vi "DiffDriveTrainSim_New_Mass_MOI.vi"(5 "j_KgM2":dbl=1.0, 6 "MeasurementStdDev":T1, 7 "Mass_Kg":dbl, 8 "WheelRadius_M":dbl, 9 "TrackWidth_M":dbl, 10 "Gearing":dbl=1.0, 11 "DriveMotor":T2 {"Kt_NMPerAmp" format="%13.5p"; "Kv_RadPerSecPerVolt" format="%13.5p"; "R_Ohms" format="%13.5p"; "FreeSpeed_RadPerSec" format="%13.5p"; "FreeCurrent_Amps" format="%13.5p"; "StallCurrent_Amps" format="%13.5p"; "StallTorque_NM" format="%13.5p"; "nominalVoltage_Volts" format="%13.5p"}) -> (0 "Size Coerced":bool, 3 "DiffDriveTrainSim":T3 {"m_Motor"."Kt_NMPerAmp" format="%13.5p"; "m_Motor"."Kv_RadPerSecPerVolt" format="%13.5p"; "m_Motor"."R_Ohms" format="%13.5p"; "m_Motor"."FreeSpeed_RadPerSec" format="%13.5p"; "m_Motor"."FreeCurrent_Amps" format="%13.5p"; "m_Motor"."StallCurrent_Amps" format="%13.5p"; "m_Motor"."StallTorque_NM" format="%13.5p"; "m_Motor"."nominalVoltage_Volts" format="%13.5p"})   [LabVIEW 2019, in "Trajectory_Library.lvlib"]
doc: "Creates a new LINEAR SYSTEM data cluster with the specified values. \n\n\nInputs: \n - XXX -- XXX.\n\nOutputs:\n - XXX -- XXX."
uses:
  Trajectory_Library.lvlib
  DIFF_DRIVE_TRAIN_SIM.ctl
  LINEAR_SYSTEM.ctl
  <vilib>/Analysis/Matrix/Datatypes/RealMatrix.ctl
  DCMOTOR.CTL
  MatBuilder_Create.vi
  MatBuilder_Fill.vi
  MatrixHelper_Zero.vi
  LinearSystem_New.vi
  <vilib>/Analysis/Matrix/NI_Matrix.lvlib
panel:
  # "<1, 1>"
  # "<States, 1>"
  # "<Outputs, 1>"
  # "<Inputs, 1>"
  # "<Outputs, 1>"
  # "<States,States>"
  # "<States,Inputs>"
  # "<Outputs,States>"
  # "<Outputs,Inputs>"
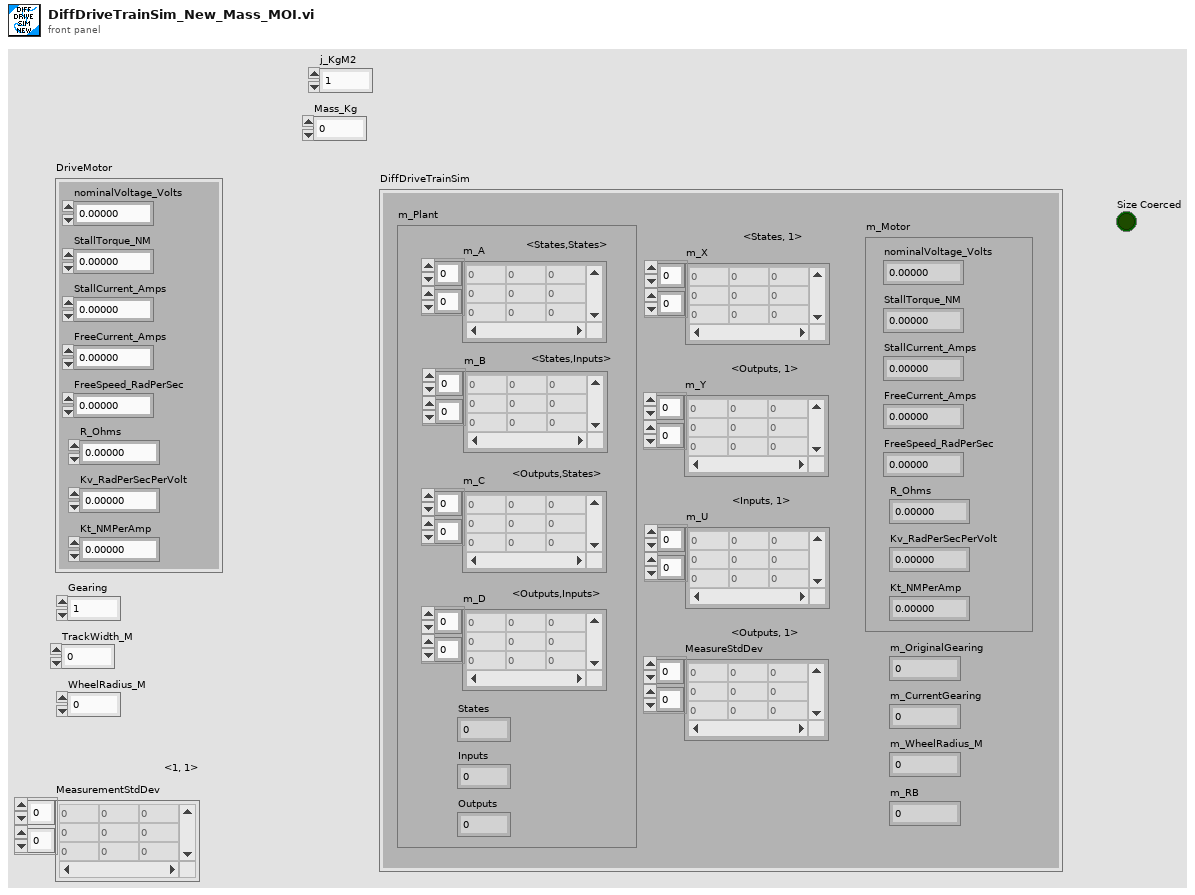
[diagram p1: front panel]
types:
  T1 = typedef "NI_Matrix.lvlib/RealMatrix.ctl" = dbl[][]
  T2 = typedef "Trajectory_Library.lvlib/DCMOTOR.CTL" = cluster{"nominalVoltage_Volts":dbl, "StallTorque_NM":dbl, "StallCurrent_Amps":dbl, "FreeCurrent_Amps":dbl, "FreeSpeed_RadPerSec":dbl, "R_Ohms":dbl, "Kv_RadPerSecPerVolt":dbl, "Kt_NMPerAmp":dbl}
  T3 = typedef "Trajectory_Library.lvlib/DIFF_DRIVE_TRAIN_SIM.ctl" = cluster{"m_Plant":T4, "m_X":T1, "m_Y":T1, "m_U":T1, "MeasureStdDev":T1, "m_Motor":T2, "m_OriginalGearing":dbl, "m_CurrentGearing":dbl, "m_WheelRadius_M":dbl, "m_RB":dbl}
  T4 = typedef "Trajectory_Library.lvlib/LINEAR_SYSTEM.ctl" = cluster{"m_A":T1, "m_B":T1, "m_C":T1, "m_D":T1, "States":i32, "Inputs":i32, "Outputs":i32}
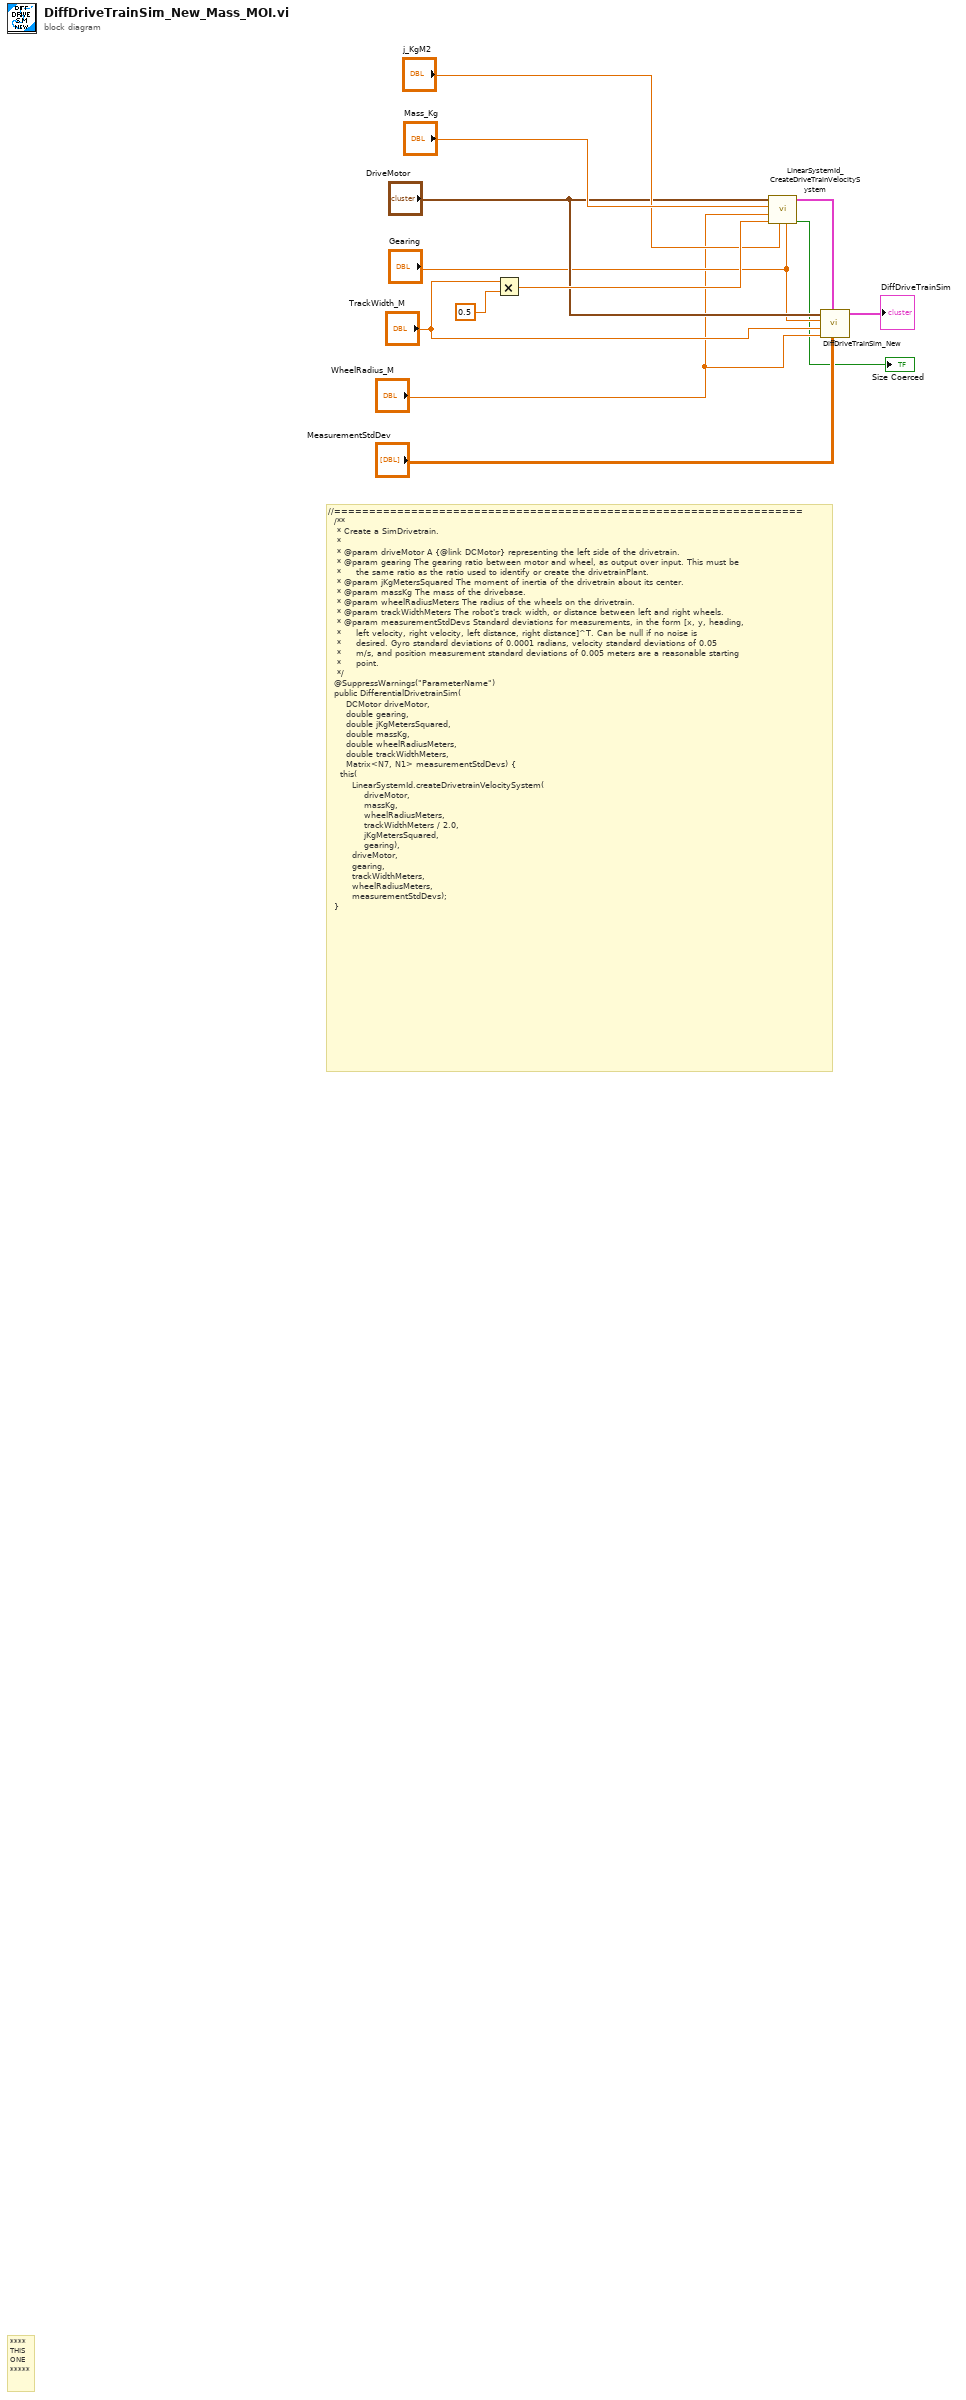
[diagram p0: block diagram]
diagram:
  # "//===================================================================\n  /**\n   * Create a SimDrivetrain.\n   *\n   * @param driveMotor A {@link DCMotor} representing the left side of the drivetrain.\n   * @param gearing The gearing ratio between motor and wheel, as output over input. This must be\n   *     the same ratio as the ratio used to identify or create the drivetrainPlant.\n   * @param jKgMetersSquared The moment of inertia of the drivetrain about its center.\n   * @param massKg The mass of the drivebase.\n   * @param wheelRadiusMeters The radius of the wheels on the drivetrain.\n   * @param trackWidthMeters The robot's track width, or distance between left and right wheels.\n   * @param measurementStdDevs Standard deviations for measurements, in the form [x, y, heading,\n   *     left velocity, right velocity, left distance, right distance]^T. Can be null if no noise is\n   *     desired. Gyro standard deviations of 0.0001 radians, velocity standard deviations of 0.05\n   *     m/s, and position measurement standard deviations of 0.005 meters are a reasonable starting\n   *     point.\n   */\n  @SuppressWarnings(\"ParameterName\")\n  public DifferentialDrivetrainSim(\n      DCMotor driveMotor,\n      double gearing,\n      double jKgMetersSquared,\n      double massKg,\n      double wheelRadiusMeters,\n      double trackWidthMeters,\n      Matrix<N7, N1> measurementStdDevs) {\n    this(\n        LinearSystemId.createDrivetrainVelocitySystem(\n            driveMotor,\n            massKg,\n            wheelRadiusMeters,\n            trackWidthMeters / 2.0,\n            jKgMetersSquared,\n            gearing),\n        driveMotor,\n        gearing,\n        trackWidthMeters,\n        wheelRadiusMeters,\n        measurementStdDevs);\n  }"
  # "****\nTHIS\nONE\n*****"
  n1 = Multiply(x="TrackWidth_M", y=0.5) -> (x*y=w9:dbl)
  n2 = call "LinearSystemId_CreateDriveTrainVelocitySystem.vi"("G"="Gearing", "JKgMetersSquared"="j_KgM2", "rbMeters"=w9, "rMeters"="WheelRadius_M", "MassKg"="Mass_Kg", "Motor"="DriveMotor") -> ("Size Coerced"=→"Size Coerced":bool, "Linearsystem"=w11:T4)  [unwired: 4 in]
  n3 = call "DiffDriveTrainSim_New.vi"("MeasurementStdDev"="MeasurementStdDev", "DriveTrainPlant"=w11, "WheelRadius_M"="WheelRadius_M", "TrackWidth_M"="TrackWidth_M", "Gearing"="Gearing", "DriveMotor"="DriveMotor") -> ("DiffDriveTrainSim"=→"DiffDriveTrainSim":T3)  [unwired: 5 in]
